vi "synnax client open.vi"(6 "error in":errorcluster, 7 "clock_skew_threshold (1s)":dbl=1.0, 8 "max_retries (3)":u32=3, 9 "Connection Config":T1={"host"="localhost", "port"=9090, "username"="synnax", "password"="seldon", "secure (False)"=FALSE, "ca_cert_file"=path "", "client_cert_file"=path "", "client_key_file"=path ""}) -> (0 "error out":errorcluster, 3 "client out":u64)   [LabVIEW 2026, in "synnax_clib.lvlib" / "Synnax Client.lvclass"]
doc: "SYNNAX_EXPORT int32_t synnax_client_open(\n const char *host,\n uint16_t port,\n const char *username,\n const char *password,\n int32_t secure,\n const char *ca_cert_file,\n SynnaxClient *out_client,\n SynnaxError err\n);"
uses:
  Synnax Client.lvclass
  typedefs/connection_config.ctl
  synnax_clib.lvlib
  synnax_clib.dll
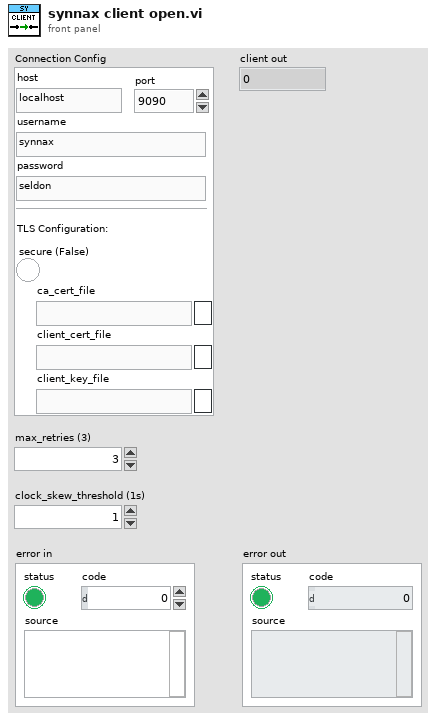
[diagram p1: front panel]
types:
  T1 = typedef "synnax_clib.lvlib/connection_config.ctl" = cluster{"host":string, "port":u16, "username":string, "password":string, "secure (False)":bool, "ca_cert_file":path, "client_cert_file":path, "client_key_file":path}
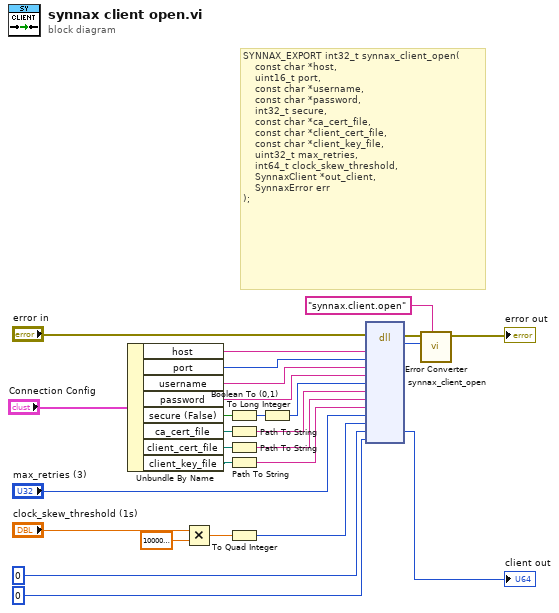
[diagram p0: block diagram]
diagram:
  # "SYNNAX_EXPORT int32_t synnax_client_open(\n    const char *host,\n    uint16_t port,\n    const char *username,\n    const char *password,\n    int32_t secure,\n    const char *ca_cert_file,\n    const char *client_cert_file,\n    const char *client_key_file,\n    uint32_t max_retries,\n    int64_t clock_skew_threshold,\n    SynnaxClient *out_client,\n    SynnaxError err\n);"
  n1 = Unbundle By Name("Connection Config") -> ("host"=w18:string, "port"=w17:u16, "username"=w16:string, "password"=w15:string, "secure (False)"=w13:bool, "ca_cert_file"=w14:path, "client_cert_file"=w12:path, "client_key_file"=w11:path)
  n2 = Multiply(x="clock_skew_threshold (1s)", y=1000000000.0) -> (x*y=w4:dbl)
  n3 = Boolean To (0,1)(Boolean=w13) -> (0, 1=w24:i16)
  n4 = Path To String(path=w14) -> (string=w10:string)
  n5 = Path To String(path=w12) -> (string=w9:string)
  n6 = Path To String(path=w11) -> (string=w8:string)
  n7 = To Quad Integer(1:w4) -> (0:w1:i64)
  n8 = To Long Integer(number=w24) -> (32bit integer=w21:i32)
  n9 = dll-call lib="C/synnax/client/labview/synnax_clib.*" fn="synnax_client_open"(error in="error in", "host"=w18, "port"=w17, "username"=w16, "password"=w15, "secure"=w21, "ca_cert_file"=w10, "client_cert_file"=w9, "client_key_file"=w8, "max_retries"="max_retries (3)", "clock_skew_threshold"=w1, "out_client"=u64 0, "err"=u64 0) -> (error out=w23:errorcluster, "return type"=w22:i32, "out_client"=→"client out":u64)  [unwired: 13 in, 1 out]
  n10 = call "Error Converter.vi"("source"="synnax.client.open", "error code"=w22, "error in (no error)"=w23) -> ("error out"=→"error out":errorcluster)  [unwired: 8 in]
